vi "parse version string.vi"(11 "full version":string) -> (0 "Fix":u32, 1 "Minor":u32, 2 "Major":u32, 3 "major.minor version":string)   [LabVIEW 2013, in "NISE_CEF_serializable configuration.lvclass"]
doc: "Strips any version information after the major and minor version numbers. This is intended to be used by <b>from string.vi</b>, as data changes should result in a major or minor version number change."
uses:
  NISE_CEF_serializable configuration.lvclass
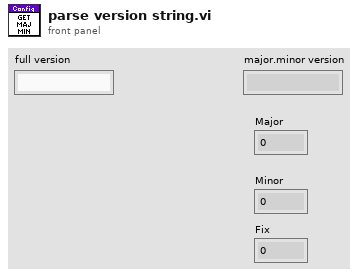
[diagram p1: front panel]
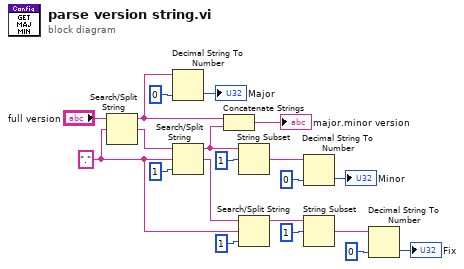
[diagram p0: block diagram]
diagram:
  w14 = "." ("search string/char (-)")
  n1 = Search/Split String(string="full version", search string/char (-)=w14) -> (substring before match=w7:string, match + rest of string=w19:string)  [unwired: 1 in, 1 out]
  n2 = Decimal String To Number(string=w7, default (0L)=u32 0 ("Major 2")) -> (number=→"Major":u32)  [unwired: 1 in, 1 out]
  n3 = Search/Split String(string=w19, search string/char (-)=w14, offset (0)=1) -> (substring before match=w6:string, match + rest of string=w15:string)  [unwired: 1 out]
  n4 = Concatenate Strings(w7, w6) -> (→"major.minor version":string)
  n5 = String Subset(string=w6, offset (0)=1) -> (substring=w4:string)  [unwired: 1 in]
  n6 = Search/Split String(string=w15, search string/char (-)=w14, offset (0)=1) -> (substring before match=w2:string)  [unwired: 2 out]
  n7 = Decimal String To Number(string=w4, default (0L)=u32 0 ("Major 2")) -> (number=→"Minor":u32)  [unwired: 1 in, 1 out]
  n8 = String Subset(string=w2, offset (0)=1) -> (substring=w1:string)  [unwired: 1 in]
  n9 = Decimal String To Number(string=w1, default (0L)=u32 0 ("Major 2")) -> (number=→"Fix":u32)  [unwired: 1 in, 1 out]
